vi "RT Host Interleaving.vi"() -> ()   [LabVIEW 2010]
uses:
  <vilib>/LabVIEW Targets/FPGA/cRIO/shared/nicrio_ModuleControls/nicrio_cRIO-9233_DataRatesRing.ctl
  <vilib>/userDefined/High Color/nirio_resource_hc.ctl
  <vilib>/rvi/interface/nirviOpenFPGA/nirviOpenFPGA.xnode
  FPGA Bitfiles/InterleavedDMA_FPGATarget_FPGAInterleaving_14DC4B3F.lvbitx
  FPGA Interleaving.vi
  <vilib>/rvi/ClientSDK/nirviWhatTheDeviceIsDoing.ctl
  <vilib>/rvi/interface/nirviMethod/nirviMethod.xnode
  <vilib>/rvi/interface/nirviReadWriteControl/nirviReadWriteControl.xnode
  <vilib>/rvi/interface/common/niFpgaNodeNameForErrorReporting.ctl
  <vilib>/rvi/errors/niLvFpgaWhatHappensToTopLevelVI.ctl
  <vilib>/rvi/interface/nirviCloseFPGA/nirviCloseFPGA.xnode
  <vilib>/FPGAPlugInAG/cRIO-9074/niLvFpga_Open_cRIO-9074.vi
  <vilib>/FPGAPlugInAG/cRIO-9074/niLvFpga_Reset_cRIO-9074.vi
  <vilib>/Utility/error.llb/Error Cluster From Error Code.vi
  <vilib>/rvi/errors/niLvFpgaAdjustHostInterfaceError.vi
  <vilib>/FPGAPlugInAG/cRIO-9074/niLvFpga_Close_cRIO-9074.vi
  NiFpgaLv.dll
panel:
  in  "Samples per Channel":i32=10
  in  "Data Rate":T1=2 items=["50.000 kS/s (NI 9233)"=2, "33.333 kS/s (NI 9233)"=3, "25.000 kS/s (NI 9233)"=34, "16.667 kS/s (NI 9233)"=35, "12.500 kS/s (NI 9233)"=36, "10.000 kS/s (NI 9233)"=37, "  8.333 kS/s (NI 9233)"=38, "  7.143 kS/s (NI 9233)"=39, "  6.250 kS/s (NI 9233)"=40, "  5.556 kS/s (NI 9233)"=41, "  5.000 kS/s (NI 9233)"=42, "  4.545 kS/s (NI 9233)"=43, "  4.167 kS/s (NI 9233)"=44, "  3.846 kS/s (NI 9233)"=45, "  3.571 kS/s (NI 9233)"=46, "  3.333 kS/s (NI 9233)"=47, "  3.125 kS/s (NI 9233)"=48, "  2.941 kS/s (NI 9233)"=49, "  2.778 kS/s (NI 9233)"=50, "  2.632 kS/s (NI 9233)"=51, "  2.500 kS/s (NI 9233)"=52, "  2.381 kS/s (NI 9233)"=53, "  2.273 kS/s (NI 9233)"=54, "  2.174 kS/s (NI 9233)"=55, "  2.083 kS/s (NI 9233)"=56, "  2.000 kS/s (NI 9233)"=57]
  out "Accelerometer Data":dbl[][](graph)
  out "Overflow Occurred?":bool
  out "Thermocouple Data":dbl[][](graph)
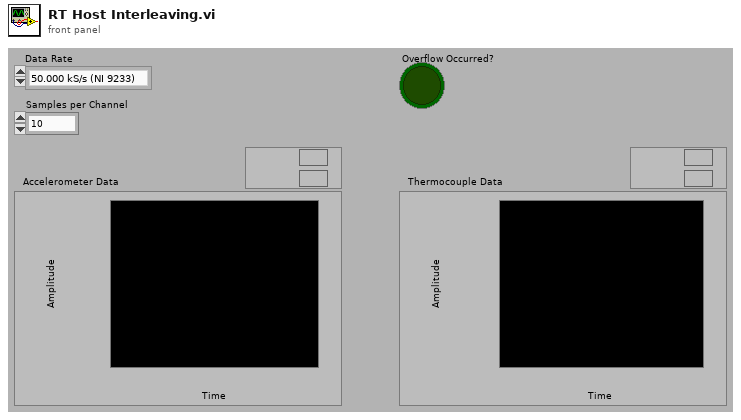
[diagram p1: front panel]
types:
  T1 = typedef "nicrio_cRIO-9233_DataRatesRing.ctl" = u8
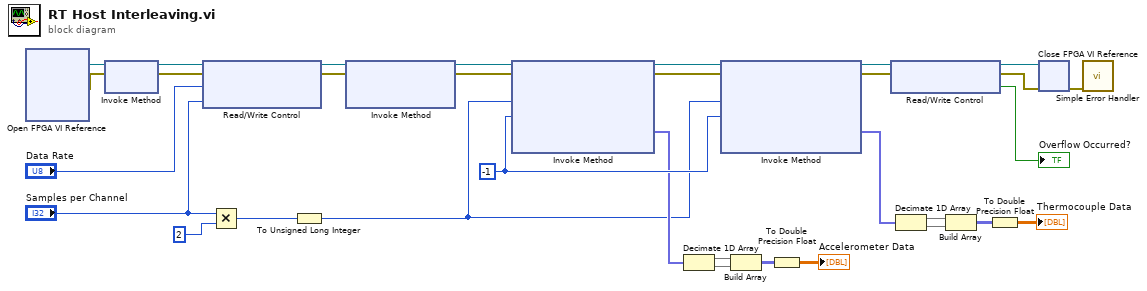
[diagram p0: block diagram]
diagram:
  w25 = -1 ("Timeout (ms)")
  n1 = xnode "Open FPGA VI Reference"() -> ("FPGA VI Reference Out"=w11:refnum<k20>, "error out"=w2:errorcluster)  [unwired: 2 in]
  n2 = xnode "Invoke Method"("FPGA VI Reference In"=w11, "error in"=w2) -> ("FPGA VI Reference Out"=w3:refnum<k20>, "error out"=w1:errorcluster)
  n3 = xnode "Read/Write Control"("FPGA VI Reference In"=w3, "error in"=w1, "Data Rate"="Data Rate", "Samples per Channel"="Samples per Channel") -> ("FPGA VI Reference Out"=w19:refnum<k20>, "error out"=w10:errorcluster)
  n4 = Multiply(x="Samples per Channel", y=2 ("Samples per Channel")) -> (x*y=w9:i32)
  n5 = To Unsigned Long Integer(number=w9) -> (unsigned 32bit integer=w8:u32)
  n6 = xnode "Invoke Method"("FPGA VI Reference In"=w19, "error in"=w10) -> ("FPGA VI Reference Out"=w16:refnum<k20>, "error out"=w14:errorcluster)  [unwired: 1 in]
  n7 = xnode "Invoke Method"("FPGA VI Reference In"=w16, "error in"=w14, "Number of Elements"=w8, "Timeout (ms)"=w25) -> ("FPGA VI Reference Out"=w15:refnum<k20>, "error out"=w13:errorcluster, "Data"=w22:fxp<+/-,24,4>[])  [unwired: 1 out]
  n8 = Decimate 1D Array(w22) -> (w24:fxp<+/-,24,4>[], w23:fxp<+/-,24,4>[])
  n9 = xnode "Invoke Method"("FPGA VI Reference In"=w15, "error in"=w13, "Number of Elements"=w8, "Timeout (ms)"=w25) -> ("FPGA VI Reference Out"=w29:refnum<k20>, "error out"=w28:errorcluster, "Data"=w21:fxp<+/-,24,-2>[])  [unwired: 1 out]
  n10 = Build Array(w24, w23) -> (w5:fxp<+/-,24,4>[][])
  n11 = To Double Precision Float(number=w5) -> (double precision float=→"Accelerometer Data":dbl[][])
  n12 = xnode "Read/Write Control"("FPGA VI Reference In"=w29, "error in"=w28) -> ("FPGA VI Reference Out"=w32:refnum<k20>, "error out"=w31:errorcluster, "Overflow Occurred"=→"Overflow Occurred?":bool)
  n13 = Decimate 1D Array(w21) -> (w27:fxp<+/-,24,-2>[], w26:fxp<+/-,24,-2>[])
  n14 = Build Array(w27, w26) -> (w7:fxp<+/-,24,-2>[][])
  n15 = To Double Precision Float(number=w7) -> (double precision float=→"Thermocouple Data":dbl[][])
  n16 = xnode "Close FPGA VI Reference"("FPGA VI Reference In"=w32, "error in"=w31) -> ("error out"=w30:errorcluster)
  n17 = call <vilib>:"Simple Error Handler.vi"("error in (no error)"=w30) -> ()  [unwired: 4 in, 5 out]
